vi "BuildVIPackage.vi"   [LabVIEW 2021]
uses:
  <vilib>/Wiresmith Technology/G CLI/CLI Class/CLI.lvclass
  <vilib>/JKI/VIPM API/VIPM API_vipm_api.lvlib
types:
  T1 = enum32{"Invalid", "Standard", "Closed", "Hidden", "Minimized", "Maximized"}
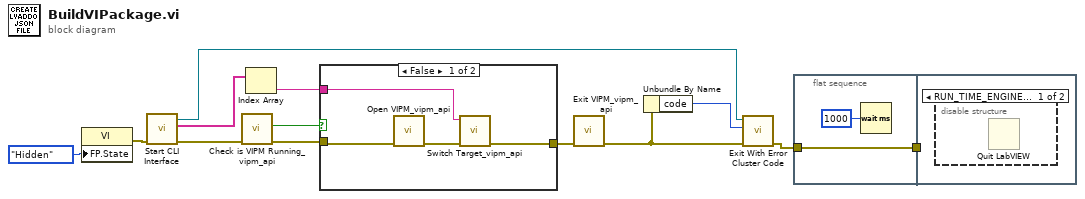
[diagram p0: block diagram]
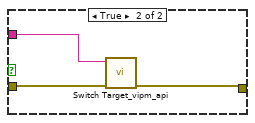
[diagram p3: hidden frame]
diagram:
  n1 = property class="VI"("FP.State"=T1."Hidden" ("Front Panel Window:State")) -> (error out=w12:errorcluster)  [unwired: 2 in, 1 out]
  n2 = call <vilib>:"Start CLI Interface.vi"("error in (no error)"=w12) -> ("error out"=w10:errorcluster, "Custom Parameters"=w7:string[], "CLI out"=w11:refnum<class "CLI.lvclass">)  [unwired: 7 in, 1 out]
  n3 = call <vilib>:"Check is VIPM Running_vipm_api.vi"("error in (no error)"=w10) -> ("error out"=w9:errorcluster, "is Running"=w8:bool)  [unwired: 9 in]
  n4 = Index Array(array=w7) -> (element=w6:string)  [unwired: 1 in]
  n5 = case shown="False" w8 {
    tunnel: w9 -> [w17 w20]
    tunnel: w6 -> [w15 w19]
    tunnel: [w14 w18] -> w2
    frame False {
      n6 = call <vilib>:"Open VIPM_vipm_api.vi"("error in (no error)"=w17) -> ("error out"=w16:errorcluster)  [unwired: 10 in]
      n7 = call <vilib>:"Switch Target_vipm_api.vi"("error in (no error)"=w16, "LabVIEW Version"=w15) -> ("error out"=w14:errorcluster)  [unwired: 9 in]
    }
    frame True {
      n8 = call <vilib>:"Switch Target_vipm_api.vi"("error in (no error)"=w20, "LabVIEW Version"=w19) -> ("error out"=w18:errorcluster)  [unwired: 9 in]
    }
  }
  n9 = call <vilib>:"Exit VIPM_vipm_api.vi"("error in (no error)"=w2) -> ("error out"=w1:errorcluster)  [unwired: 10 in]
  n10 = Unbundle By Name(w1) -> ("code"=w3:i32)
  n11 = call <vilib>:"Exit With Error Cluster Code.vi"("error in (no error)"=w1, "No Error Code (0)"=w3, "CLI in"=w11) -> ("error out"=w4:errorcluster)  [unwired: 8 in]
  n12 = flat-sequence {
    tunnel: w4 -> [w22]
    tunnel: [w22] -> w5
    tunnel: w5 -> [_]
    frame #0 {
      n13 = Wait (ms)(milliseconds to wait=u32 1000) -> ()  [unwired: 1 out]
    }
    frame #1 {
      n14 = disable-structure shown="RUN_TIME_ENGINE==True" {
        frame condition #0 {
          n15 = Quit LabVIEW() -> ()  [unwired: 1 in]
        }
        frame condition #1 (active) {
        }
      }
    }
  }
